vi "Update Plot.vi"(4 "Good fit?":dbl[](array[numeric]) format="%#_4p", 6 "Peak Plot":cluster{"Ramp Pattern":dbl[], "X":dbl[]}[](array[cluster]), 8 "error in (no error)":errorcluster, 9 "Plots":cluster{"X":dbl[], "Array":dbl[]}[](array[cluster]), 10 "Best fit results":dbl[][](array[numeric]) format="%#_4p", 11 "Resonance Detector in":refnum<class "Resonance Detector.lvclass">) -> (0 "error out":errorcluster, 3 "Resonance Detector out":refnum<class "Resonance Detector.lvclass">)   [LabVIEW 2016, in "Resonance Detector.lvclass"]
uses:
  Resonance Detector.lvclass
  Resonance Detector.lvclass/Resonance Detector.ctl
panel:
  # "F0         dF     Ampl   Phase   Xbgrd   Ybgrd"
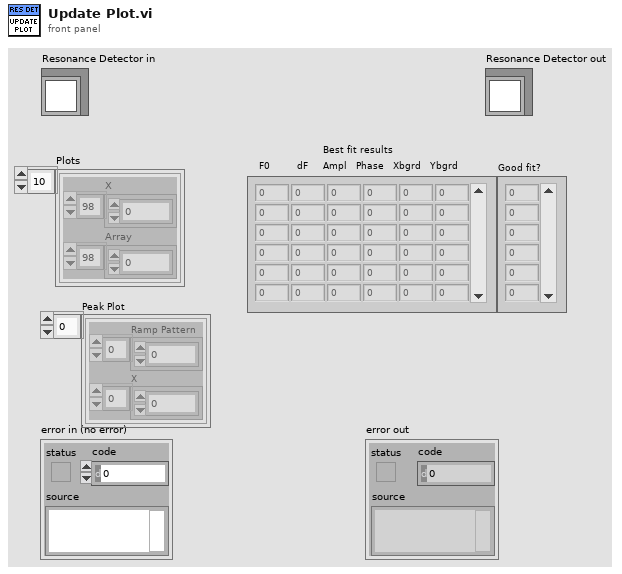
[diagram p1: front panel]
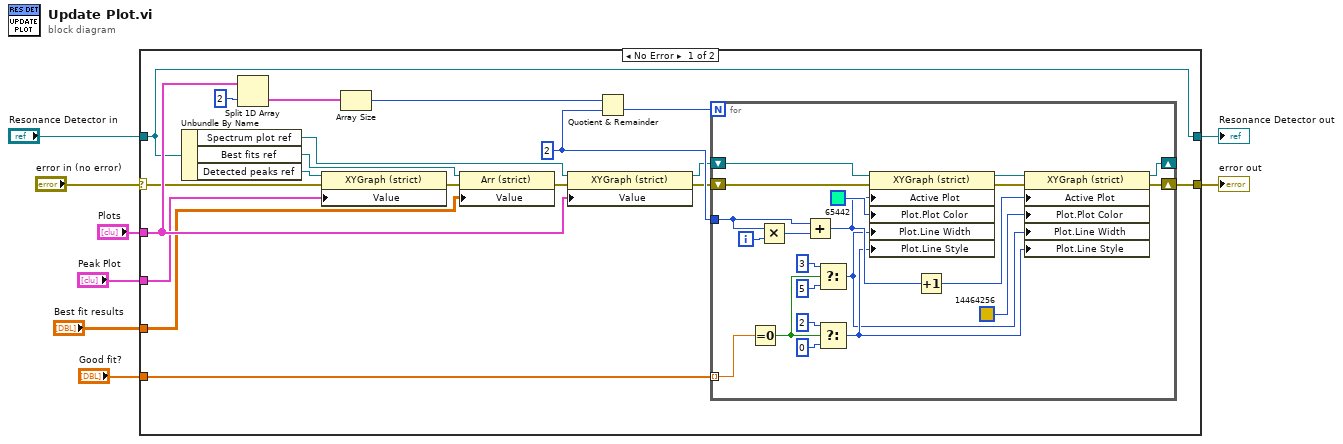
[diagram p0: block diagram]
diagram:
  n1 = case shown="No Error" "error in (no error)" {
    selector: "error in (no error)" -> [w14 w50]
    tunnel: [w10 w50] -> w7
    tunnel: [w13 w49] -> w5
    tunnel: "Resonance Detector in" -> [w13 w49]
    tunnel: "Plots" -> [w15 _]
    tunnel: "Best fit results" -> [w12 _]
    tunnel: "Peak Plot" -> [w11 _]
    tunnel: "Good fit?" -> [w9 _]
    frame No Error {
      w27 = 2 ("y")
      n2 = Unbundle By Name(w13) -> ("Spectrum plot ref"=w21:refnum<vi>, "Best fits ref"=w17:refnum<vi>, "Detected peaks ref"=w16:refnum<vi>)
      n3 = Split 1D Array(array=w15, index=2) -> (second subarray=w20:cluster{"X":dbl[], "Array":dbl[]}[])  [unwired: 1 out]
      n4 = property class="XYGraph (strict)"(reference=w16, error in=w14, "Value"=w11) -> (error out=w18:errorcluster)  [unwired: 1 out]
      n5 = Array Size(array=w20) -> (size(s)=w25:i32)
      n6 = property class="Arr (strict)"(reference=w17, error in=w18, "Value"=w12) -> (error out=w22:errorcluster)  [unwired: 1 out]
      n7 = property class="XYGraph (strict)"(reference=w21, error in=w22, "Value"=w15) -> (reference out=w24:refnum<vi>, error out=w23:errorcluster)
      n8 = Quotient & Remainder(x=w25, y=w27) -> (floor(x/y)=w26:i32)  [unwired: 1 out]
      n9 = for {
        N: w26 -> [_]
        shift-right: [w39] -> w10
        shift-left: w23 -> [w47]
        shift-right: [w38] -> _
        shift-left: w24 -> [w48]
        tunnel: w27 -> [w36]
        tunnel: w9 -> [w35] mode=indexing
        i -> [w46]
        n10 = Equal To 0?(x=w35) -> (x = 0?=w29:bool)
        n11 = Multiply(x=w36, y=w46) -> (x*y=w37:i32)
        n12 = Add(x=w36, y=w37) -> (x+y=w42:i32)
        n13 = Select(t=u8 3 ("Plot.Line Width"), s=w29, f=u8 5 ("Plot.Line Width")) -> (s? t:f=w28:u8)
        n14 = Select(t=u8 2, s=w29, f=u8 0 ("Plot.Line Style")) -> (s? t:f=w33:u8)
        n15 = property class="XYGraph (strict)"(reference=w48, error in=w47, "Active Plot"=w42, "Plot.Plot Color"=u32 65442 ("Color Box"), "Plot.Line Width"=w28, "Plot.Line Style"=w33) -> (reference out=w44:refnum<vi>, error out=w43:errorcluster)
        n16 = Increment(x=w42) -> (x+1=w41:i32)
        n17 = property class="XYGraph (strict)"(reference=w44, error in=w43, "Active Plot"=w41, "Plot.Plot Color"=u32 14464256 ("Color Box"), "Plot.Line Width"=w28, "Plot.Line Style"=w33) -> (reference out=w38:refnum<vi>, error out=w39:errorcluster)
      }
    }
    frame Error {
    }
  }
  "error out" <- w7
  "Resonance Detector out" <- w5
